vi "Read Config File.vi"(8 "error in (no error)":errorcluster, 11 "Front Panel Menu in":refnum<class "Front Panel Menu.lvclass">) -> (0 "error out":errorcluster, 2 "Ref":T1, 3 "Front Panel Menu out":refnum<class "Front Panel Menu.lvclass">)   [LabVIEW 2024, in "Front Panel Menu.lvclass"]
uses:
  Front Panel Menu.lvclass
  <vilib>/Utility/config.llb/Config Data RefNum.ctl
  Type Def/Menu Item Group.ctl
  Type Def/Menu Item.ctl
  Front Panel Menu.lvclass/Front Panel Menu.ctl
  <vilib>/Utility/config.llb/Read Key (String).vi
  Ancestor Class/Actor/System Actor/System Actor.lvclass
  <vilib>/Utility/config.llb/NI_LVConfig.lvlib
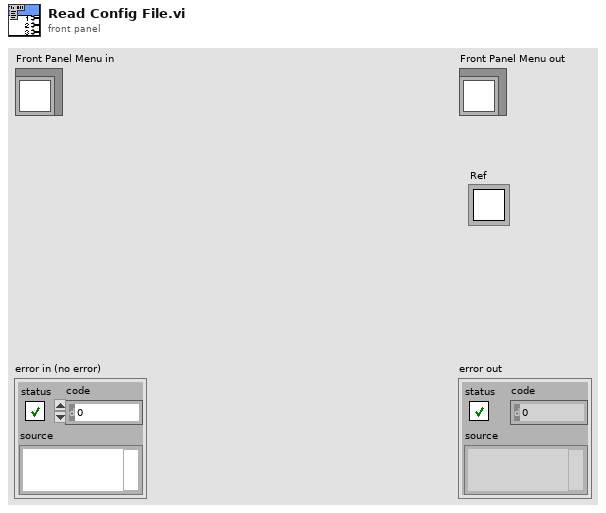
[diagram p1: front panel]
types:
  T1 = typedef "NI_LVConfig.lvlib/Config Data RefNum.ctl" = refnum<k1>
  T2 = typedef "Menu Item Group.ctl" = cluster{"Array":T3[]}[]
  T3 = typedef "Menu Item.ctl" = cluster{"Parent Node Index":i32, "Item":string}
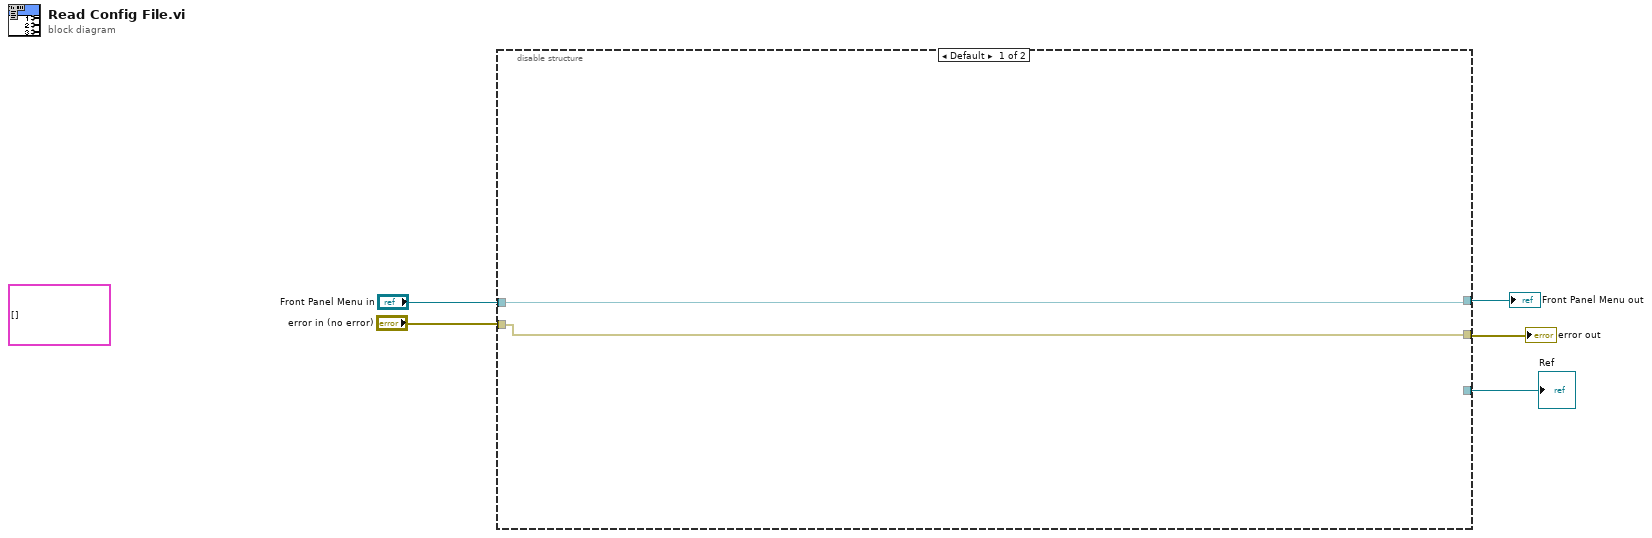
[diagram p0: block diagram]
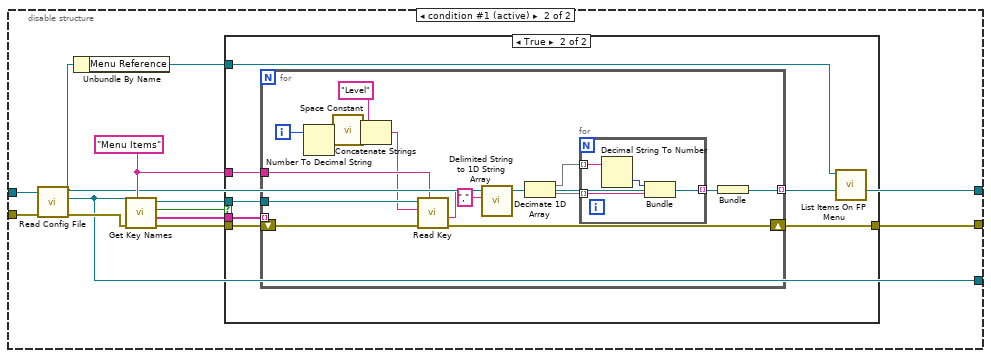
[diagram p2: hidden frame]
diagram:
  (unwired) T2 [] ("Menu Items")
  n1 = disable-structure shown="Default" {
    disable-tunnel: "error in (no error)" -> [w6 w12]
    disable-tunnel: "Front Panel Menu in" -> [w7 w11]
    disable-tunnel: [w6 w10] -> w3
    disable-tunnel: [_ w9] -> w2
    disable-tunnel: [w7 w8] -> w1
    frame condition #0 {
    }
    frame condition #1 (active) {
      w13 = "Menu Items" ("section")
      n2 = call-parent "Read Config File.vi"("error in (no error)"=w12, "System Actor in"=w11) -> ("error out"=w15:errorcluster, "Ref"=w9:T1, "System Actor out"=w8:refnum<class "Front Panel Menu.lvclass">)  [unwired: 7 in]
      n3 = Unbundle By Name(w8) -> ("Menu Reference"=w19:refnum<k9>)
      n4 = call <vilib>:"Get Key Names.vi"("section"=w13, "error in (no error)"=w15, "refnum"=w9) -> ("error out"=w16:errorcluster, "key names"=w17:string[], "section exists?"=w18:bool, "refnum out"=w14:T1)  [unwired: 5 in]
      n5 = case shown="True" w18 {
        tunnel: [w20 w27] -> w10
        tunnel: w14 -> [_ w26]
        tunnel: w16 -> [w20 w25]
        tunnel: w17 -> [_ w24]
        tunnel: w13 -> [_ w23]
        tunnel: w19 -> [_ w21]
        frame False {
        }
        frame True {
          n6 = for {
            shift-right: [w35] -> w27
            shift-left: w25 -> [w38]
            tunnel: w26 -> [w39]
            tunnel: w24 -> [_] mode=indexing
            tunnel: w23 -> [w37]
            tunnel: [w28] -> w22 mode=indexing
            i -> [w43]
            n7 = Number To Decimal String(number=w43) -> (decimal integer string=w42:string)  [unwired: 1 in]
            n8 = call <vilib>:"Space Constant.vi"() -> ("String"=w41:string)
            n9 = Concatenate Strings("Level" ("string"), w41, w42) -> (w36:string)
            n10 = call-poly <vilib>:"Read Key.vi"("section"=w37, "error in (no error)"=w38, "key"=w36, "refnum"=w39) -> ("error out"=w35:errorcluster, "value"=w34:string)  [unwired: 4 in, 2 out]
            n11 = call <vilib>:"Delimited String to 1D String Array.vi"("delimiter"=",", "delimited string"=w34) -> ("string array"=w32:string[])  [unwired: 9 in]
            n12 = Decimate 1D Array(w32) -> (w31:string[], w30:string[])
            n13 = for {
              tunnel: w31 -> [w47] mode=indexing
              tunnel: w30 -> [w46] mode=indexing
              tunnel: [w44] -> w29 mode=indexing
              n14 = Decimal String To Number(string=w47) -> (number=w45:i32)  [unwired: 2 in, 1 out]
              n15 = Bundle(w45, "String"=w46) -> (w44:cluster{i32, "String":string})  [unwired: 1 in]
            }
            n16 = Bundle(w29) -> (w28:cluster{cluster{i32, "String":string}[]})  [unwired: 1 in]
          }
          n17 = call "List Items On FP Menu.vi"("Item Groups In"=w22, "Menu Reference"=w21) -> ()  [unwired: 10 in]
        }
      }
    }
  }
  "error out" <- w3
  "Front Panel Menu out" <- w1
  "Ref" <- w2
